vi "Send ADC.vi"(8 "error in (no error)":errorcluster, 9 "Channel":u8, 10 "VISA resource name":refnum<visa-resource-name>, 11 "Arduino in":refnum<class "Arduino.lvclass">) -> (0 "error out":errorcluster, 1 "Response":i32, 2 "VISA resource name 2":refnum<visa-resource-name>, 3 "Arduino out":refnum<class "Arduino.lvclass">)   [LabVIEW 2020, in "Arduino.lvclass"]
uses:
  Arduino.lvclass
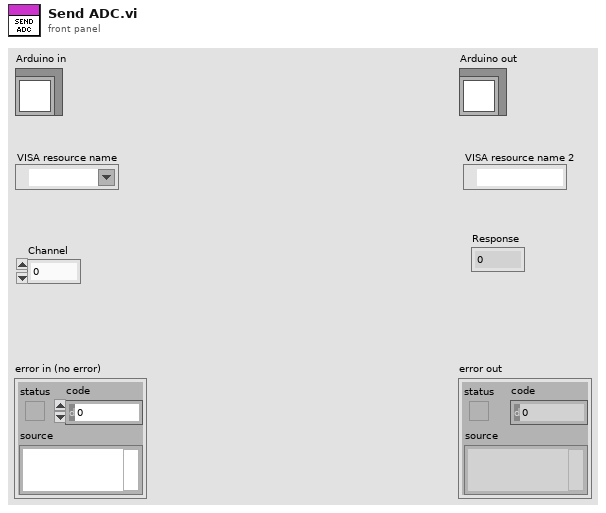
[diagram p1: front panel]
types:
  T1 = enum16{"Write", "Read", "Config", "Reset", "Close"}
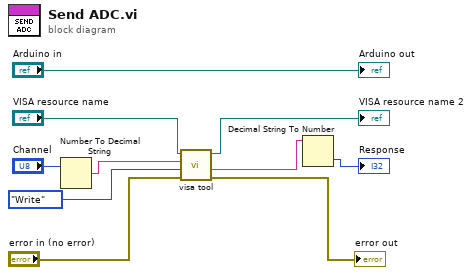
[diagram p0: block diagram]
diagram:
  n1 = Number To Decimal String(number="Channel") -> (decimal integer string=w5:string)  [unwired: 1 in]
  n2 = call "visa tool.vi"("error in (no error)"="error in (no error)", "Opciones"=T1."Write", "Write"=w5, "VISA com port"="VISA resource name") -> ("error out"=→"error out":errorcluster, "Read"=w2:string, "VISA com port 2"=→"VISA resource name 2":refnum<visa-resource-name>)  [unwired: 5 in]
  n3 = Decimal String To Number(string=w2) -> (number=→"Response":i32)  [unwired: 2 in, 1 out]
  "Arduino out" <- "Arduino in"
